vi "Get SubVI Terminal (by Name).vi"(8 "error in (no error)":errorcluster, 10 "Terminal name":string, 11 "SubVI in":refnum<vi>) -> (0 "error out":errorcluster, 1 "Found?":bool, 2 "SubVI Term ref":refnum<vi>, 3 "SubVI out":refnum<vi>)   [LabVIEW 2019, in "gRPC Template Creation Utility.lvlib"]
uses:
  gRPC Template Creation Utility.lvlib
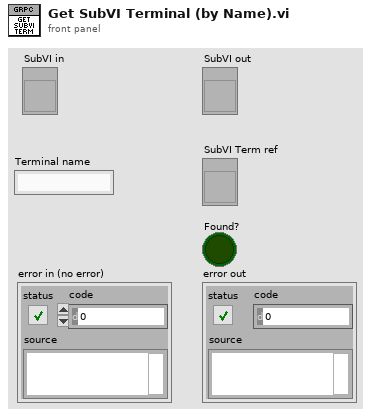
[diagram p1: front panel]
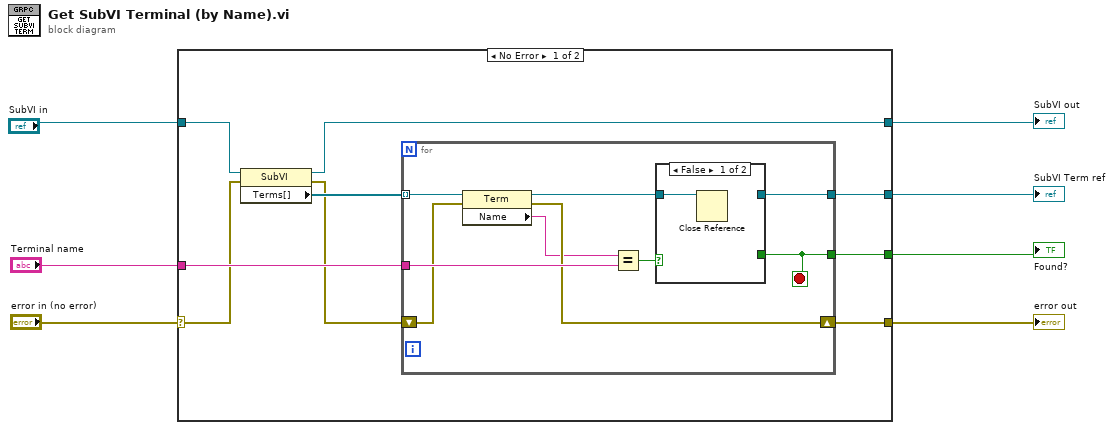
[diagram p0: block diagram]
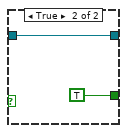
[diagram p2: hidden frame]
diagram:
  n1 = case shown="No Error" "error in (no error)" {
    selector: "error in (no error)" -> [w10 w30]
    tunnel: "Terminal name" -> [w16 _]
    tunnel: [w8 w30] -> w6
    tunnel: "SubVI in" -> [w14 w29]
    tunnel: [w11 w29] -> w2
    tunnel: [w15 _] -> w4
    tunnel: [w12 _] -> w1
    frame No Error {
      n2 = property class="SubVI"(reference=w14, error in=w10) -> (reference out=w11:refnum<vi>, error out=w9:errorcluster, "Terms[]"=w13:refnum<vi>[])
      n3 = for {
        tunnel: w16 -> [w25]
        tunnel: [w23] -> w15
        tunnel: w13 -> [w22] mode=indexing
        tunnel: [w20] -> w12
        shift-right: [w18] -> w8
        shift-left: w9 -> [w19]
        stop <- w23 stop-if-true
        n4 = property class="Term"(reference=w22, error in=w19) -> (reference out=w21:refnum<vi>, error out=w18:errorcluster, "Name"=w17:string)
        n5 = Equal?(x=w17, y=w25) -> (x = y?=w24:bool)
        n6 = case shown="False" w24 {
          tunnel: [_ TRUE] -> w23
          tunnel: w21 -> [w26 w27]
          tunnel: [_ w27] -> w20
          frame False {
            n7 = Close Reference(reference=w26) -> ()  [unwired: 1 in, 1 out]
          }
          frame True {
          }
        }
      }
    }
    frame Error {
    }
  }
  "error out" <- w6
  "Found?" <- w4
  "SubVI out" <- w2
  "SubVI Term ref" <- w1
